vi "F5xxx_pq_load_preset.vi"(7 "channel":enum16{"PRI", "SEC"}(ring), 8 "error in":errorcluster, 10 "preset name":string, 11 "VISA in":refnum<visa-resource-name>) -> (0 "error out":errorcluster, 3 "VISA out":refnum<visa-resource-name>)   [LabVIEW 2013]
uses:
  Fluke 5XXX Series Multicalibrators.lvlib
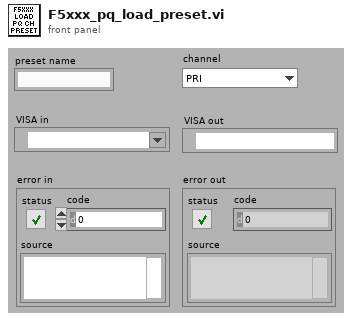
[diagram p1: front panel]
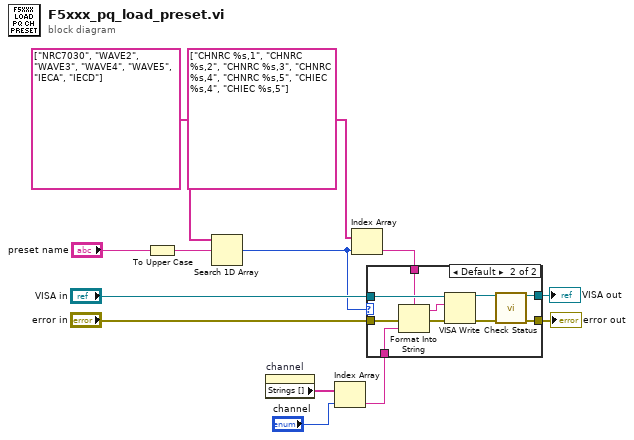
[diagram p0: block diagram]
diagram:
  n1 = To Upper Case(1:"preset name") -> (0:w5:string)
  n2 = Search 1D Array(1D array=string[] ["NRC7030", "WAVE2", "WAVE3", "WAVE4", "WAVE5", "IECA", "IECD"], element=w5) -> (index of element=w1:i32)  [unwired: 1 in]
  n3 = property on="channel" class="Enum (strict)"() -> ("Strings []"=w10:string[])  [unwired: 2 in, 2 out]
  n4 = Index Array(array=w10, index="channel") -> (element=w2:string)
  n5 = Index Array(array=string[] ["CHNRC %s,1", "CHNRC %s,2", "CHNRC %s,3", "CHNRC %s,4", "CHNRC %s,5", "CHIEC %s,4", "CHIEC %s,5"], index=w1) -> (element=w3:string)
  n6 = case shown="Default" w1 {
    tunnel: "VISA in" -> [w14 w25]
    tunnel: [w15 w22] -> w12
    tunnel: [w14 w21] -> w11
    tunnel: "error in" -> [w15 w18]
    tunnel: w3 -> [_ w17]
    tunnel: w2 -> [_ w16]
    frame -1 {
    }
    frame Default {
      n7 = Format Into String(format string=w17, error in=w18, w16) -> (resulting string=w19:string, error out=w20:errorcluster)  [unwired: 1 in]
      n8 = VISA Write(VISA resource name=w25, write buffer=w19, error in (no error)=w20) -> (VISA resource name out=w23:refnum<visa-resource-name>, error out=w24:errorcluster)  [unwired: 1 out]
      n9 = call "Check Status.vi"("VISA resource name"=w23, "error in (no error)"=w24) -> ("VISA resource name out"=w21:refnum<visa-resource-name>, "error out"=w22:errorcluster)  [unwired: 12 in]
    }
  }
  "error out" <- w12
  "VISA out" <- w11
